vi "Append XY Arrays.vi"(8 "error in (no error)":errorcluster, 10 "XY [] B in":cluster{"X-array":dbl[], "Y-array":dbl[]}[](array[cluster]), 11 "XY [] A in":cluster{dbl[], dbl[]}[](array[cluster])) -> (0 "error out":errorcluster, 3 "XY [] out":cluster{dbl[], dbl[]}[](array[cluster]))   [LabVIEW 2016, in "Transport.lvclass"]
uses:
  Transport.lvclass
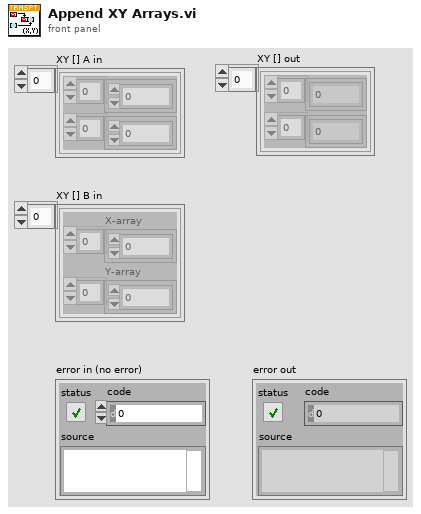
[diagram p1: front panel]
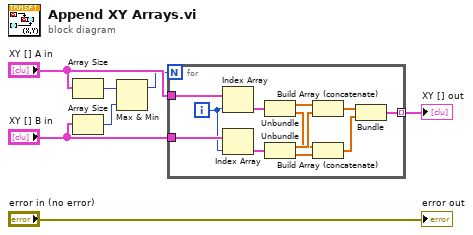
[diagram p0: block diagram]
diagram:
  n1 = Array Size(array="XY [] A in") -> (size(s)=w3:i32)
  n2 = Array Size(array="XY [] B in") -> (size(s)=w2:i32)
  n3 = Max & Min(x=w3, y=w2) -> (max(x,y)=w1:i32)  [unwired: 1 out]
  n4 = for {
    N: w1 -> [_]
    tunnel: "XY [] A in" -> [w10]
    tunnel: "XY [] B in" -> [w18]
    tunnel: [w12] -> w7 mode=indexing
    i -> [w9]
    n5 = Index Array(array=w10, index=w9) -> (element=w8:cluster{dbl[], dbl[]})
    n6 = Index Array(array=w18, index=w9) -> (element=w11:cluster{"X-array":dbl[], "Y-array":dbl[]})
    n7 = Unbundle(w8) -> (w19:dbl[], w15:dbl[])
    n8 = Unbundle(w11) -> ("X-array"=w17:dbl[], "Y-array"=w14:dbl[])
    n9 = Build Array (concatenate)(w19, w17) -> (w16:dbl[])
    n10 = Build Array (concatenate)(w15, w14) -> (w13:dbl[])
    n11 = Bundle(w16, w13) -> (w12:cluster{dbl[], dbl[]})  [unwired: 1 in]
  }
  "XY [] out" <- w7
  "error out" <- "error in (no error)"
